vi "Write Message Box.vi"(5 "Message Box":refnum<class "MessageBox.lvclass">, 9 "RasPi Compiler in":refnum<class "RasPi Compiler.lvclass">) -> (3 "RasPi Compiler out":refnum<class "RasPi Compiler.lvclass">)   [LabVIEW 2014, in "RasPi Compiler.lvclass"]
uses:
  RasPi Compiler.lvclass
  RasPi_Services/MessageBox/MessageBox.lvclass
  RasPi Compiler.lvclass/RasPi Compiler.ctl
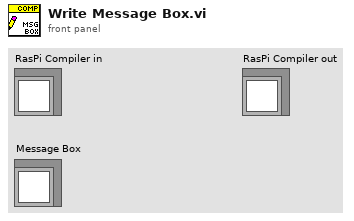
[diagram p1: front panel]
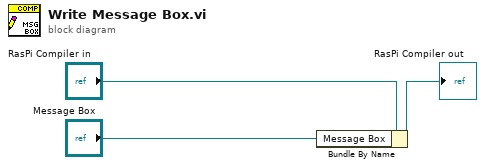
[diagram p0: block diagram]
diagram:
  n1 = Bundle By Name(cluster="RasPi Compiler in", "Message Box"="Message Box") -> (→"RasPi Compiler out":refnum<class "RasPi Compiler.lvclass">)
